vi "LS Durability Main ALTERNATE TWO(FPGA).vi"() -> ()   [LabVIEW 2013]
uses:
  <vilib>/rvi/Emulation/niFpgaSctlEmulationGetInTimedLoop.vi
  <vilib>/rvi/Emulation/niFpgaEmulationReportErrorSimple.vi
  <vilib>/rvi/Emulation/niFpgaGetClockAttributes.vi
  <vilib>/rvi/eio/common/nirviEmuTemplateMethod_errors.vi
  <vilib>/rvi/Emulation/niFpgaCriticalErrorInLSC.vi
  <vilib>/eio/EIONode/EIONode.xnode
panel:
  out "Bankvalid":bool
  out "Open":bool
  out "Opens Detected":i16[](array[numeric])
  in  "Opens Resets":bool[](array[boolean])=[FALSE, FALSE, FALSE, FALSE, FALSE, FALSE, FALSE, FALSE, FALSE, FALSE, FALSE, FALSE]
  in  "Enable Opens":bool[](array[boolean])=[FALSE, FALSE, FALSE, FALSE, FALSE, FALSE, FALSE, FALSE, FALSE, FALSE, FALSE, FALSE]
  out "AI Loop Time (usec)":u32=70
  out "Analog Inputs":fxp<+/-,28,17>[](array[numeric])
  in  "Enable Readings":bool[](array[boolean])=[FALSE, FALSE, FALSE, FALSE, FALSE, FALSE, FALSE, FALSE, FALSE, FALSE, FALSE, FALSE]
  out "Bank2Active":bool
  in  "Bank2(Pulse/Const)":bool
  in  "Bank2Const(On/Off)":bool
  out "Bank2On":bool
  out "Bank1Active":bool
  in  "(S)Enable Opens":bool
  in  "(S)Opens Resets":bool
  out "(S)Opens Detected":i16
  out "Bank1On":bool
  out "Opens Loop Time (usec)":u32=1000
  in  "Bank1Const(On/Off)":bool
  in  "Bank1(Pulse/Const)":bool
  in  "PWM Period (Ticks)":u32=4000000
  in  "Duty (Ticks)":i32=2000000
  in  "Invert PWM?":bool=TRUE
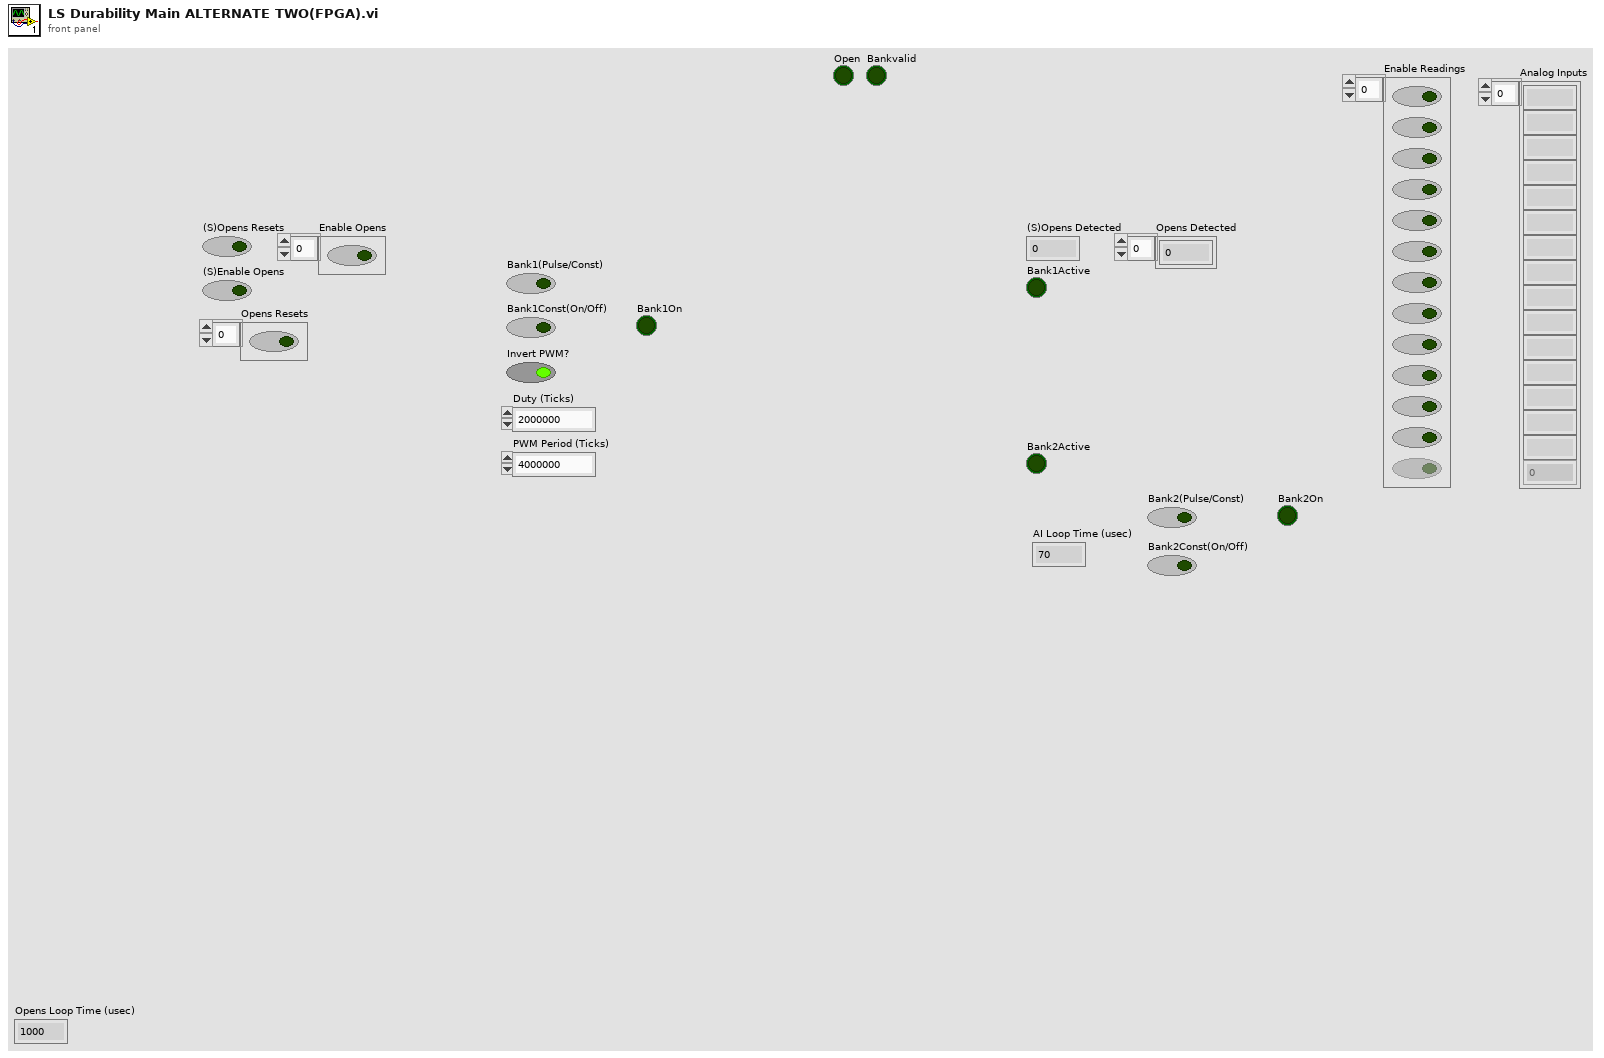
[diagram p1: front panel]
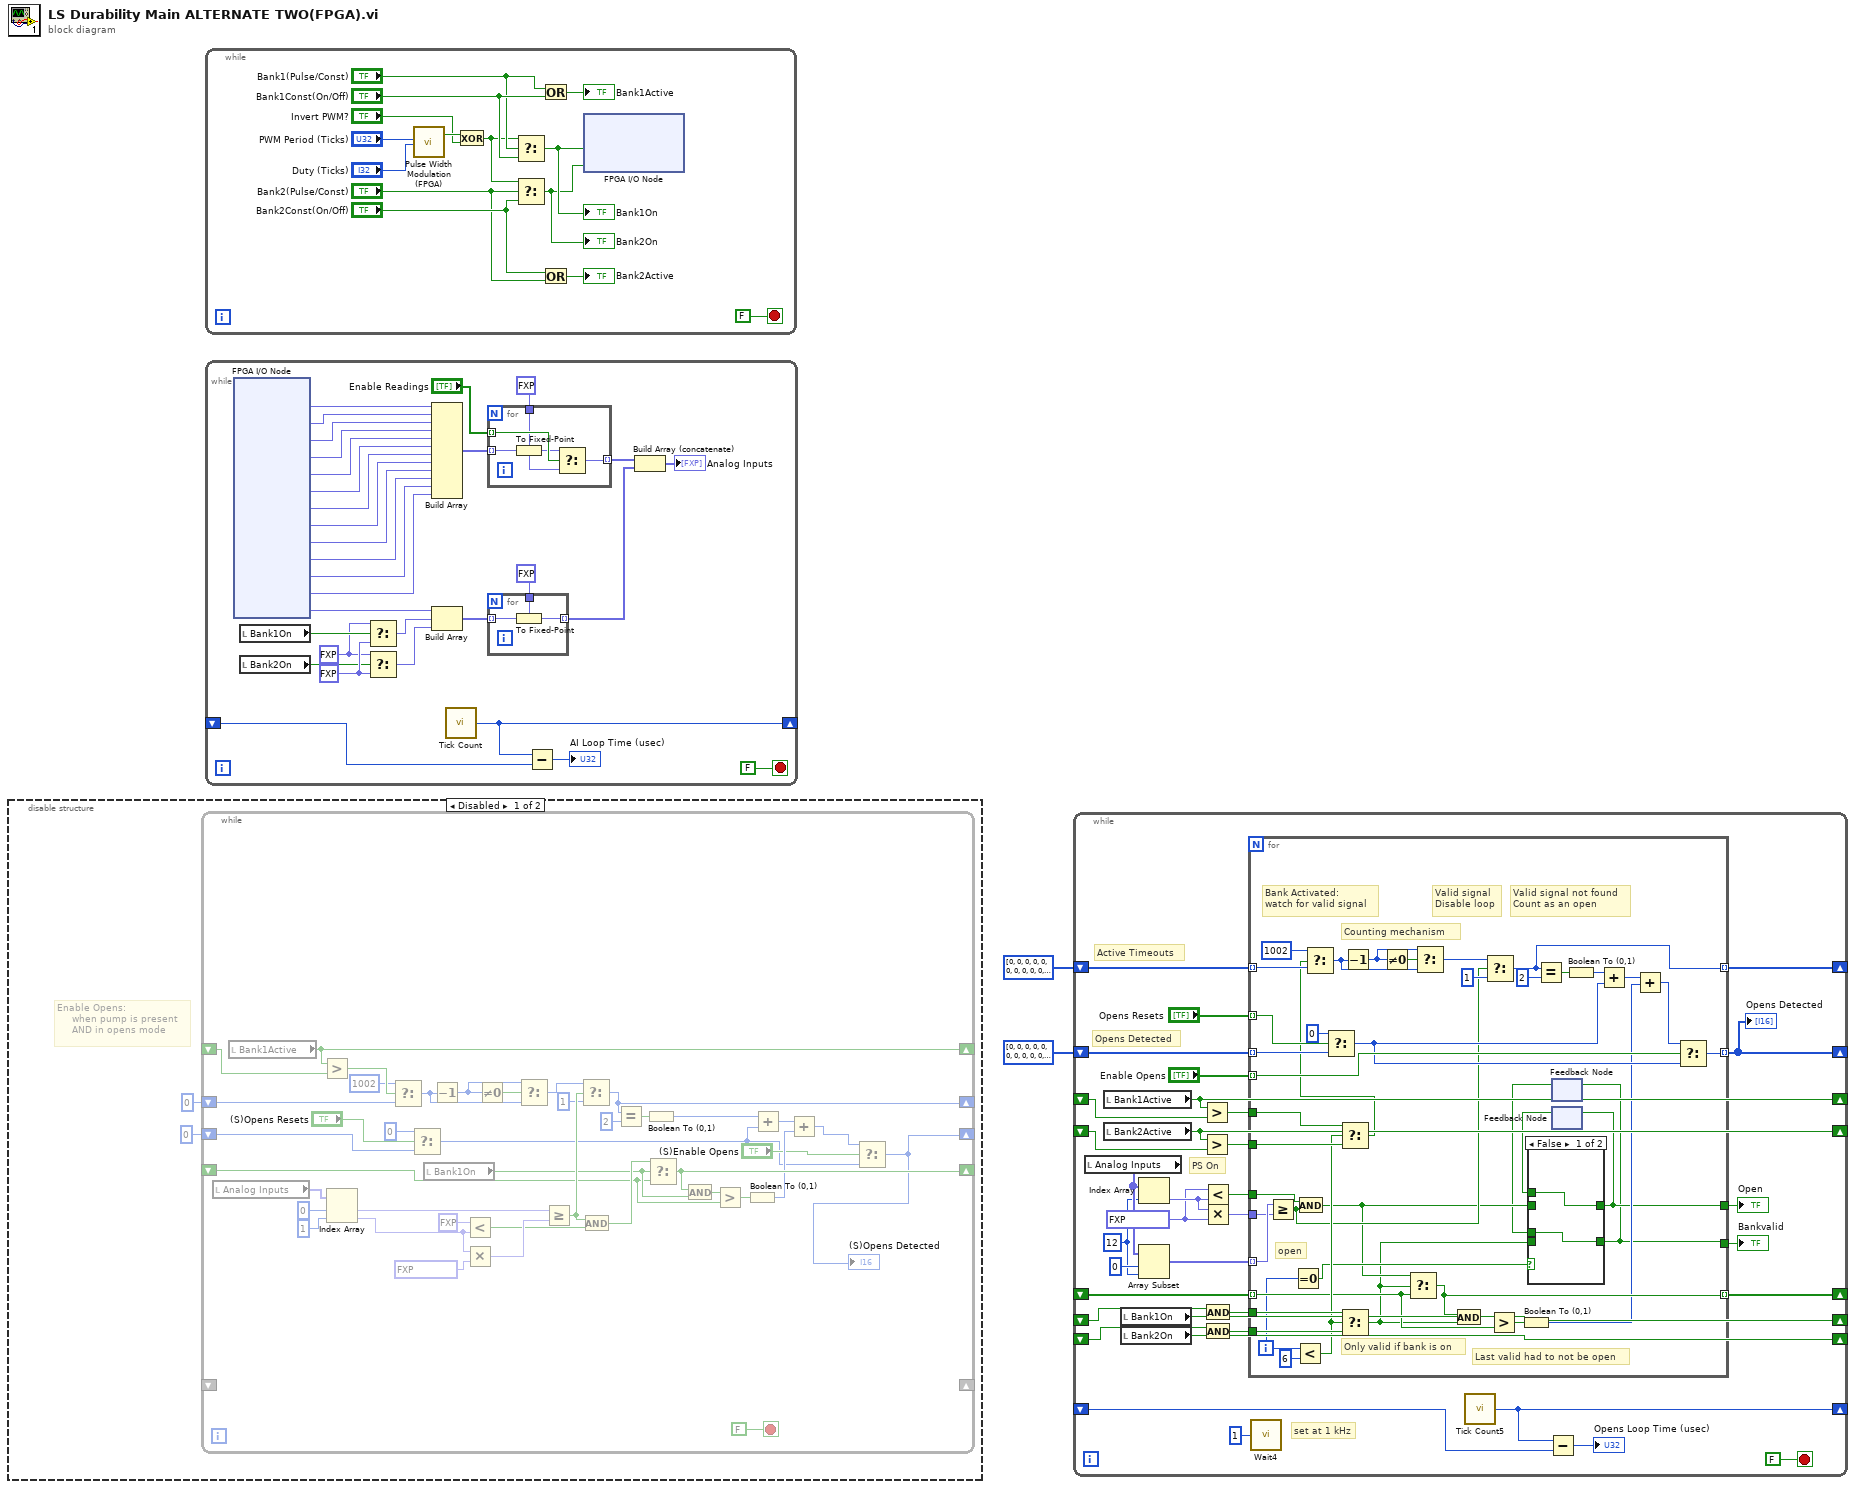
[diagram p0: block diagram]
diagram:
  n1 = disable-structure shown="Disabled" {
    frame Disabled {
      # "Enable Opens:\n     when pump is present\n     AND in opens mode"
      n2 = while {
        shift-right: _ -> [w45]
        shift-left: _ -> [w44]
        shift-right: [w43] -> _
        shift-left: _ -> [w42]
        shift-right: [w23] -> _
        shift-left: u16 0 -> [w40]
        shift-right: [w19] -> _
        shift-left: _ -> [w16]
        shift-right: [w9] -> _
        shift-left: i16 0 -> [w7]
        stop <- FALSE stop-if-true
        n3 = local read "Analog Inputs"() -> (w35:fxp<+/-,28,17>[])
        n4 = local read "Bank1Active"() -> (w43:bool)
        n5 = Greater?(x=w43, y=w42) -> (0:w41:bool)
        n6 = Index Array(array=w35, index #1=0 ("index"), index #2=1 ("index")) -> (element #1=w27:fxp<+/-,28,17>, element #2=w30:fxp<+/-,28,17>)
        n7 = Select(t=u16 1002, s=w41, f=w40) -> (s? t:f=w37:u16)
        n8 = Select(t=i16 0, s="(S)Opens Resets", f=w7) -> (s? t:f=w6:i16)
        n9 = local read "Bank1On"() -> (w18:bool)
        n10 = Decrement(x=w37) -> (x-1=w36:u16)
        n11 = Less?(x=fxp<+/-,28,17> 1.0, y=w30) -> (x < y?=w28:bool)
        n12 = Multiply(x=w30, y=fxp<+,8,0> 0.94921875) -> (x*y=w29:fxp<+/-,36,17>)
        n13 = Not Equal To 0?(x=w36) -> (x != 0?=w38:bool)
        n14 = Select(t=w36, s=w38, f=w37) -> (s? t:f=w25:u16)
        n15 = Greater Or Equal?(x=w27, y=w29) -> (x >= y?=w26:bool)
        n16 = Select(t=w25, s=w26, f=u16 1) -> (s? t:f=w23:u16)
        n17 = And(x=w26, y=w28) -> (x .and. y?=w20:bool)
        n18 = Equal?(x=w23, y=u16 2) -> (x = y?=w21:bool)
        n19 = Boolean To (0,1)(Boolean=w21) -> (0, 1=w14:i16)
        n20 = Select(t=w20, s=w18, f=w16) -> (s? t:f=w19:bool)
        n21 = And(x=w19, y=w18) -> (x .and. y?=w17:bool)
        n22 = Greater?(x=w17, y=w16) -> (0:w15:bool)
        n23 = Boolean To (0,1)(Boolean=w15) -> (0, 1=w12:i16)
        n24 = Add(x=w14, y=w6) -> (x+y=w13:i16)
        n25 = Add(x=w13, y=w12) -> (x+y=w10:i16)
        n26 = Select(t=w10, s="(S)Enable Opens", f=w6) -> (s? t:f=w9:i16)
        "(S)Opens Detected" <- w9
      }
    }
    frame Enabled {
    }
  }
  n27 = while {
    stop <- FALSE stop-if-true
    n28 = call "Pulse Width Modulation (FPGA).vi"("PWM Period (Ticks)"="PWM Period (Ticks)", "PWM Duty Cycle (Ticks)"="Duty (Ticks)") -> ("PWM DO"=w57:bool)  [unwired: 14 in, 3 out]
    n29 = Exclusive Or(1:"Invert PWM?", 2:w57) -> (0:w50:bool)
    n30 = Select(t=w50, s="Bank1(Pulse/Const)", f="Bank1Const(On/Off)") -> (s? t:f=w55:bool)
    "Bank1On" <- w55
    n31 = Select(t=w50, s="Bank2(Pulse/Const)", f="Bank2Const(On/Off)") -> (s? t:f=w51:bool)
    "Bank2On" <- w51
    n32 = Or(x="Bank1(Pulse/Const)", y="Bank1Const(On/Off)") -> (x .or. y?=→"Bank1Active":bool)
    n33 = Or(x="Bank2Const(On/Off)", y="Bank2(Pulse/Const)") -> (x .or. y?=→"Bank2Active":bool)
    n34 = xnode "FPGA I/O Node"("RMC/DIO0"=w55, "RMC/DIO1"=w51) -> ()  [unwired: 3 in, 3 out]
  }
  n35 = while {
    shift-right: [w90] -> _
    shift-left: _ -> [w89]
    stop <- FALSE stop-if-true
    w63 = fxp<+/-,24,5> 1.0 ("AI13")
    w66 = fxp<+/-,24,5> 0.0 ("AI13")
    n36 = xnode "FPGA I/O Node"() -> ("AI0"=w87:fxp<+/-,24,5>, "AI1"=w86:fxp<+/-,24,5>, "AI2"=w85:fxp<+/-,24,5>, "AI3"=w84:fxp<+/-,24,5>, "AI4"=w83:fxp<+/-,24,5>, "AI5"=w82:fxp<+/-,24,5>, "AI6"=w81:fxp<+/-,24,5>, "AI7"=w80:fxp<+/-,24,5>, "AI8"=w79:fxp<+/-,24,5>, "AI9"=w78:fxp<+/-,24,5>, "AI10"=w77:fxp<+/-,24,5>, "AI11"=w76:fxp<+/-,24,5>, "AI12"=w73:fxp<+/-,24,5>)  [unwired: 13 in, 13 out]
    n37 = local read "Bank1On"() -> (w65:bool)
    n38 = local read "Bank2On"() -> (w64:bool)
    n39 = Select(t=w63, s=w65, f=w66) -> (s? t:f=w62:fxp<+/-,24,5>)
    n40 = Select(t=w63, s=w64, f=w66) -> (s? t:f=w61:fxp<+/-,24,5>)
    n41 = Build Array(w87, w86, w85, w84, w83, w82, w81, w80, w79, w78, w77, w76) -> (w75:fxp<+/-,24,5>[])
    n42 = Build Array(w73, w62, w61) -> (w71:fxp<+/-,24,5>[])
    n43 = call "Tick Count"() -> ("Tick Count(uSec)"=w90:u32)
    n44 = for {
      tunnel: w75 -> [w99] mode=indexing
      tunnel: fxp<+/-,28,17> 0.0 ("AI0") -> [w96]
      tunnel: [w95] -> w69 mode=indexing
      tunnel: "Enable Readings" -> [w98] mode=indexing
      n45 = To Fixed-Point(fixed-point type=w96, number=w99) -> (fixed-point=w97:fxp<+/-,28,17>)
      n46 = Select(t=w97, s=w98, f=w96) -> (s? t:f=w95:fxp<+/-,28,17>)
    }
    n47 = for {
      tunnel: w71 -> [w94] mode=indexing
      tunnel: fxp<+/-,28,17> 0.0 ("AI0") -> [w93]
      tunnel: [w92] -> w70 mode=indexing
      n48 = To Fixed-Point(fixed-point type=w93, number=w94) -> (fixed-point=w92:fxp<+/-,28,17>)
    }
    n49 = Subtract(x=w90, y=w89) -> (x-y=→"AI Loop Time (usec)":u32)
    n50 = Build Array (concatenate)(w69, w70) -> (→"Analog Inputs":fxp<+/-,28,17>[])
  }
  n51 = while {
    shift-right: [w133] -> _
    shift-left: _ -> [w132]
    shift-right: [w128] -> _
    shift-left: _ -> [w127]
    shift-right: [w129] -> _
    shift-left: _ -> [w126]
    shift-right: [w109] -> _
    shift-left: u16[] [0, 0, 0, 0, 0, 0, 0, 0, 0, 0, 0, 0] -> [w122]
    shift-right: [w108] -> _
    shift-left: i16[] [0, 0, 0, 0, 0, 0, 0, 0, 0, 0, 0, 0] -> [w123]
    shift-right: [w111] -> _
    shift-left: _ -> [w110]
    shift-right: [w105] -> _
    shift-left: _ -> [w102]
    shift-right: [w104] -> _
    shift-left: _ -> [w103]
    stop <- FALSE stop-if-true
    w114 = fxp<+,8,0> 0.94921875
    w117 = 12 ("length")
    # "PS On"
    # "Active Timeouts"
    # "Opens Detected"
    # "set at 1 kHz"
    n52 = local read "Analog Inputs"() -> (w119:fxp<+/-,28,17>[])
    n53 = local read "Bank1Active"() -> (w128:bool)
    n54 = local read "Bank2Active"() -> (w129:bool)
    n55 = local read "Bank1On"() -> (w104:bool)
    n56 = local read "Bank2On"() -> (w105:bool)
    n57 = Index Array(array=w119, index=w117) -> (element=w115:fxp<+/-,28,17>)
    n58 = Array Subset(array=w119, index=0, length=w117) -> (w116:fxp<+/-,28,17>[])
    n59 = Greater?(x=w128, y=w127) -> (0:w125:bool)
    n60 = Greater?(x=w129, y=w126) -> (0:w124:bool)
    n61 = Less?(x=w114, y=w115) -> (x < y?=w112:bool)
    n62 = Multiply(x=w115, y=w114) -> (x*y=w113:fxp<+/-,36,17>)
    n63 = And(x=w103, y=w104) -> (x .and. y?=w100:bool)
    n64 = And(x=w102, y=w105) -> (x .and. y?=w101:bool)
    n65 = for {
      tunnel: w100 -> [w176]
      tunnel: w101 -> [w175]
      tunnel: w125 -> [w173]
      tunnel: w124 -> [w174]
      tunnel: w123 -> [w170] mode=indexing
      tunnel: w122 -> [w159] mode=indexing
      tunnel: "Opens Resets" -> [w169] mode=indexing
      tunnel: "Enable Opens" -> [w157] mode=indexing
      tunnel: [w154] -> w108 mode=indexing
      tunnel: w113 -> [w151]
      tunnel: w116 -> [w152] mode=indexing
      tunnel: w112 -> [w150]
      tunnel: [w149] -> w111 mode=indexing
      tunnel: w110 -> [w146] mode=indexing
      tunnel: [w144] -> w109 mode=indexing
      tunnel: [w138] -> w107
      tunnel: [w135] -> w106
      i -> [w142]
      # "Last valid had to not be open"
      # "Only valid if bank is on"
      # "open"
      # "Valid signal not found\nCount as an open"
      # "Valid signal\nDisable loop"
      # "Counting mechanism"
      # "Bank Activated:\nwatch for valid signal"
      n66 = Greater Or Equal?(x=w152, y=w151) -> (x >= y?=w143:bool)
      n67 = Equal To 0?(x=w142) -> (x = 0?=w141:bool)
      n68 = Less?(x=w142, y=6) -> (x < y?=w172:bool)
      n69 = And(x=w150, y=w143) -> (x .and. y?=w140:bool)
      n70 = Select(t=i16 0, s=w169, f=w170) -> (s? t:f=w156:i16)
      n71 = Select(t=w173, s=w172, f=w174) -> (s? t:f=w153:bool)
      n72 = Select(t=u16 1002, s=w153, f=w159) -> (s? t:f=w158:u16)
      n73 = Select(t=w176, s=w172, f=w175) -> (s? t:f=w137:bool)
      n74 = Decrement(x=w158) -> (x-1=w163:u16)
      n75 = Not Equal To 0?(x=w163) -> (x != 0?=w162:bool)
      n76 = Select(t=w140, s=w137, f=w146) -> (s? t:f=w149:bool)
      n77 = Select(t=w163, s=w162, f=w158) -> (s? t:f=w164:u16)
      n78 = And(x=w149, y=w137) -> (x .and. y?=w147:bool)
      n79 = Select(t=w164, s=w143, f=u16 1) -> (s? t:f=w144:u16)
      n80 = Greater?(x=w147, y=w146) -> (0:w148:bool)
      n81 = Boolean To (0,1)(Boolean=w148) -> (0, 1=w145:i16)
      n82 = Equal?(x=w144, y=u16 2) -> (x = y?=w166:bool)
      n83 = feedback #1() -> (w136:bool)  [unwired: 1 in]
      n84 = feedback #2() -> (w139:bool)  [unwired: 1 in]
      n85 = case shown="False" w141 {
        tunnel: w140 -> [_ w181]
        tunnel: [w179 w181] -> w138
        tunnel: w139 -> [w179 _]
        tunnel: w137 -> [_ w180]
        tunnel: [w178 w180] -> w135
        tunnel: w136 -> [w178 _]
        frame False {
        }
        frame True {
        }
      }
      n86 = feedback-in #1(w135) -> ()
      n87 = feedback-in #2(w138) -> ()
      n88 = Boolean To (0,1)(Boolean=w166) -> (0, 1=w167:i16)
      n89 = Add(x=w167, y=w156) -> (x+y=w168:i16)
      n90 = Add(x=w168, y=w145) -> (x+y=w155:i16)
      n91 = Select(t=w155, s=w157, f=w156) -> (s? t:f=w154:i16)
    }
    "Opens Detected" <- w108
    "Open" <- w107
    "Bankvalid" <- w106
    n92 = call "Wait4"("Count(mSec)"=u32 1) -> ()  [unwired: 1 out]
    n93 = call "Tick Count5"() -> ("Tick Count(uSec)"=w133:u32)
    n94 = Subtract(x=w133, y=w132) -> (x-y=→"Opens Loop Time (usec)":u32)
  }
